vi "HistoryFile.vi"() -> ()   [LabVIEW 2018]
uses:
  <vilib>/vision/Image Controls.llb/IMAQ Image.ctl
panel:
  out "激光器型号":string
  out "存储时间":string
  out "History_Spetrometer":T1
  out "History_Near/Far":T3
  out "History_Scope":T4
  out "History _PolarMeter":cluster{" 偏振方向":string, "偏振度":string}
  out "History_Power/Energy":T5
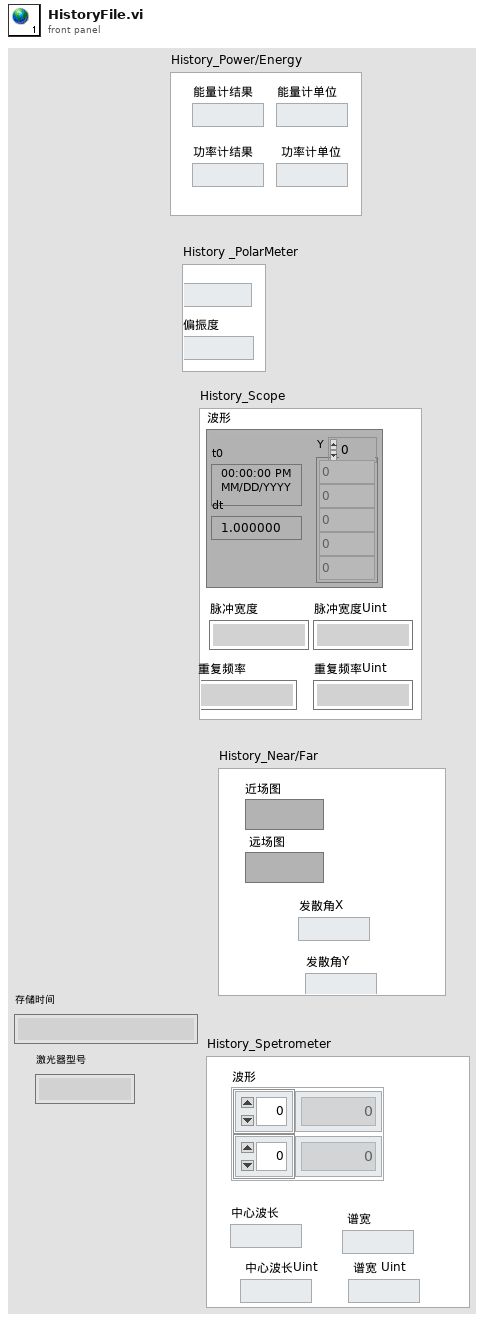
[diagram p1: front panel]
types:
  T1 = cluster{"中心波长":string, " 谱宽":string, " 中心波长Uint":string, " 谱宽 Uint":string, "波形":cluster{"数组":dbl[], "数组":dbl[]}}
  T2 = typedef "IMAQ Image.ctl" = refnum<image>
  T3 = cluster{"近场图":T2, " 远场图":T2, "发散角X":string, "发散角Y":string}
  T4 = cluster{"波形":waveform(dbl), "脉宽":string, "重频":string, "脉冲宽度Uint":string, "重复频率Uint":string}
  T5 = cluster{"能量计结果":string, "功率计结果":string, "能量计单位":string, " 功率计单位":string}
diagram:
